vi "generate_DAC_voltages_V3_justMineZtrajectoryTest.vi"(7 "focus mode?":bool, 8 "derived values":T1, 9 "scan specification":T4={"x amplitude"=0, "x resolution (pixels)"=0, "x offset fly-forward (iterations)"=0, "x offset fly-back (iterations)"=0, "y resolution (nr. of lines)"=0, "y step size"=0, "iterations per pixel"=0, "number of frames"=0, "y offset (pixels)"=0, "number of y-brake lines  (before y-fly-back)"=0, "number y-brake lines (after y-fly-back)"=0, "number of y-fly-back steps"=8, "lines per z step"=0, "number of z/intensity tuples"=0, "number of repetitions (volumes or planes)"=0, "z step size derived"=0, "choose the beginning of z scan"=FALSE, "number of frames (settings)"=0, "FPGA trajectory?"=FALSE}, 10 "counter cluster in":T2, 11 "resonant trigger":bool) -> (0 "acquire?":bool, 1 "fly-back acquisition phase?":bool, 2 "counter cluster out":T2, 3 "DAC voltages":T3 {"ch6" max=4095 step=1; "ch5" max=4095 step=1; "ch4" max=4095 step=1; "ch3" max=4095 step=1; "ch2" max=4095 step=1; "ch1" max=4095 step=1; "ch0" max=4095 step=1})   [LabVIEW 2010]
uses:
  scan_specification_cluster.ctl
  common_typedefs/DAC_voltage_cluster.ctl
  counter_cluster.ctl
  derived_values_cluster.ctl
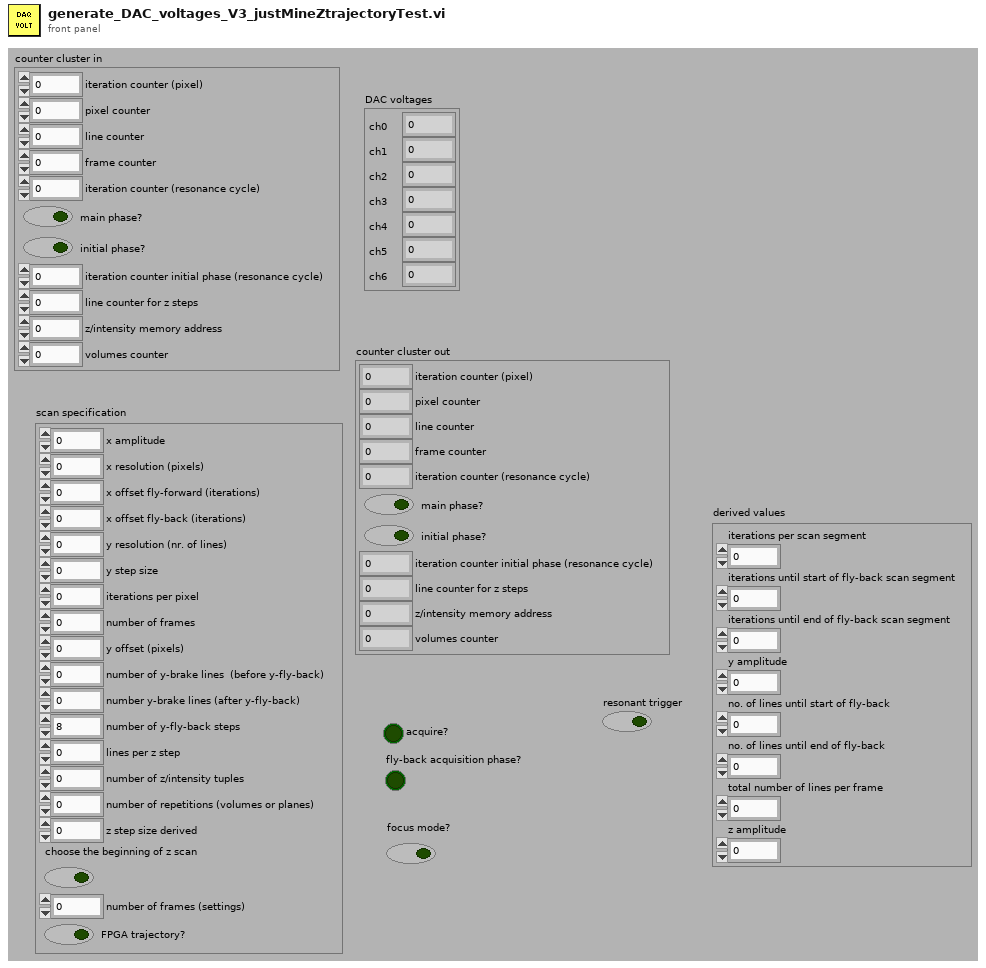
[diagram p1: front panel]
types:
  T1 = typedef "derived_values_cluster.ctl" = cluster{"iterations per scan segment":u16, "iterations until start of fly-back scan segment":u16, "iterations until end of fly-back scan segment":u16, "y amplitude":u16, "no. of lines until start of fly-back":u16, "no. of lines until end of fly-back":u16, "total number of lines per frame ":u16, "z amplitude":u16}
  T2 = typedef "counter_cluster.ctl" = cluster{"iteration counter (pixel)":u16, "pixel counter":u16, "line counter":u16, "frame counter":u16, "iteration counter (resonance cycle)":u16, "main phase?":bool, "initial phase?":bool, "iteration counter initial phase (resonance cycle)":u16, "line counter for z steps":u16, "z/intensity memory address":u32, "volumes counter":u16}
  T3 = typedef "DAC_voltage_cluster.ctl" = cluster{"ch0":u16, "ch1":i16, "ch2":i16, "ch3":u16, "ch4":u16, "ch5":u16, "ch6":u16}
  T4 = typedef "scan_specification_cluster.ctl" = cluster{"x amplitude":u16, "x resolution (pixels)":u16, "x offset fly-forward (iterations)":u16, "x offset fly-back (iterations)":u16, "y resolution (nr. of lines)":u16, "y step size":u16, "iterations per pixel":u16, "number of frames":i32, "y offset (pixels)":u16, "number of y-brake lines  (before y-fly-back)":u16, "number y-brake lines (after y-fly-back)":u16, "number of y-fly-back steps":u16, "lines per z step":u16, "number of z/intensity tuples":u16, "number of repetitions (volumes or planes)":i32, "z step size derived":u16, "choose the beginning of z scan":bool, "number of frames (settings)":i32, "FPGA trajectory?":bool}
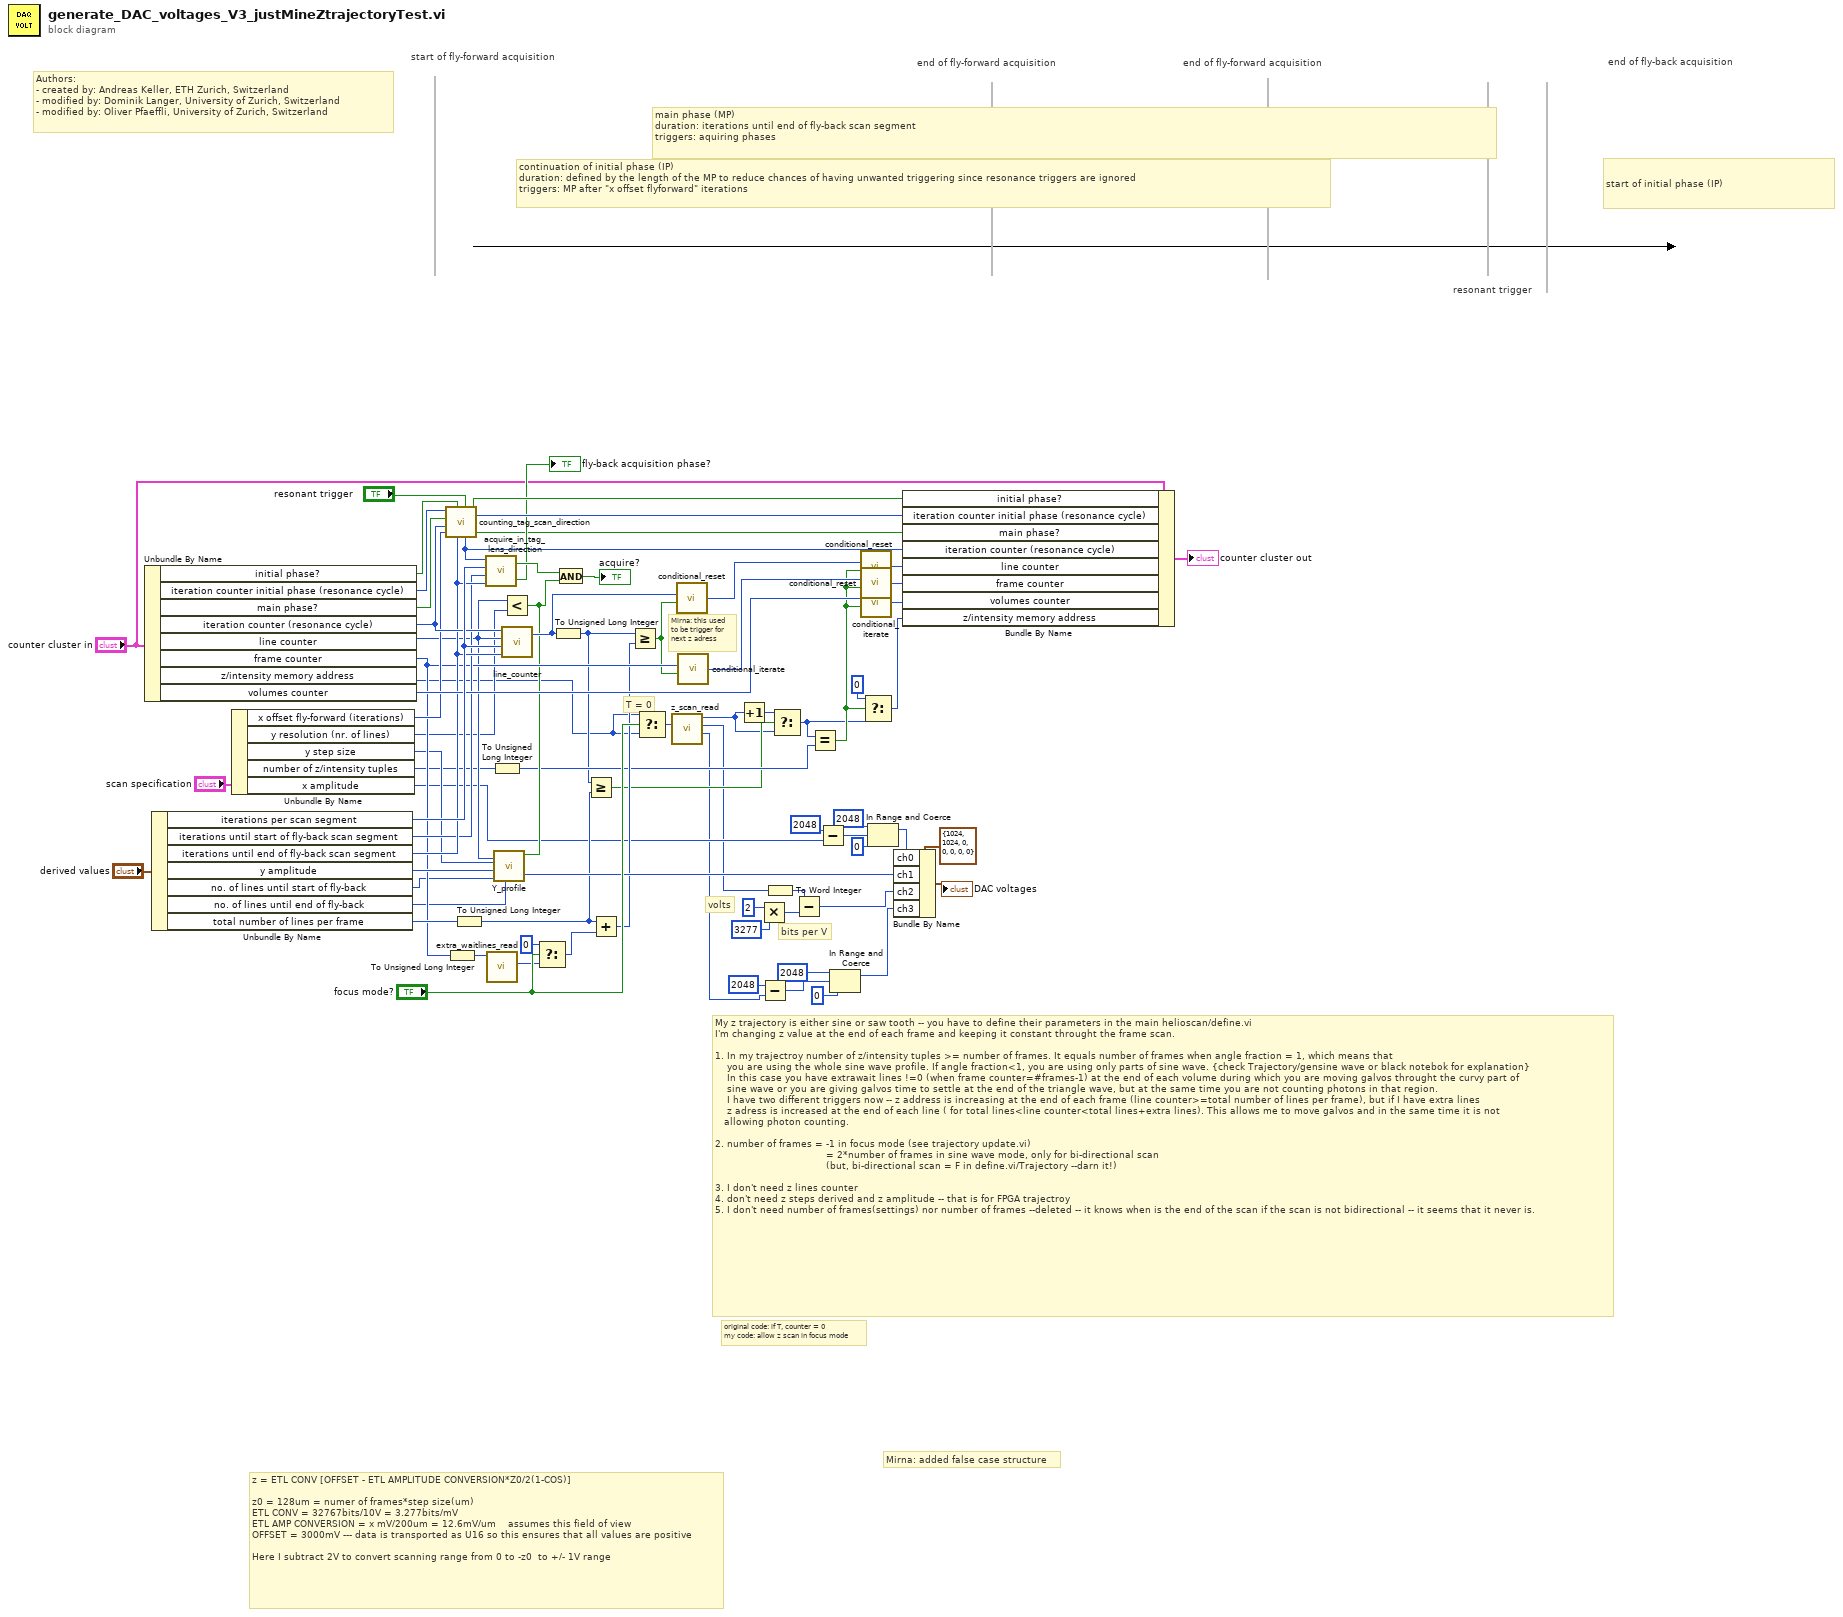
[diagram p0: block diagram]
diagram:
  # "bits per V"
  # "volts"
  # "Mirna: this used \nto be trigger for \nnext z adress"
  # "T = 0"
  # "My z trajectory is either sine or saw tooth -- you have to define their parameters in the main helioscan/define.vi\nI'm changing z value at the end of each frame and keeping it constant throught the frame scan.\n\n1. In my trajectroy number of z/intensity tuples >= number of frames. It equals number of frames when angle fraction = 1, which means that \n    you are using the whole sine wave profile. If angle fraction<1, you are using only parts of sine wave. {check Trajectory/gensine wave or black notebok for explanation}\n    In this case you have extrawait lines !=0 (when frame counter=#frames-1) at the end of each volume during which you are moving galvos throught the curvy part of\n    sine wave or you are giving galvos time to settle at the end of the triangle wave, but at the same time you are not counting photons in that region.\n    I have two different triggers now -- z address is increasing at the end of each frame (line counter>=total number of lines per frame), but if I have extra lines \n    z adress is increased at the end of each line ( for total lines<line counter<total lines+extra lines). This allows me to move galvos and in the same time it is not \n   allowing photon counting.\n   \n2. number of frames = -1 in focus mode (see trajectory update.vi)\n                                     = 2*number of frames in sine wave mode, only for bi-directional scan \n                                     (but, bi-directional scan = F in define.vi/Trajectory --darn it!)\n             \n3. I don't need z lines counter\n4. don't need z steps derived and z amplitude -- that is for FPGA trajectroy\n5. I don't need number of frames(settings) nor number of frames --deleted -- it knows when is the end of the scan if the scan is not bidirectional -- it seems that it never is."
  # "z = ETL CONV [OFFSET - ETL AMPLITUDE CONVERSION*Z0/2(1-COS)]\n\nz0 = 128um = numer of frames*step size(um)\nETL CONV = 32767bits/10V = 3.277bits/mV\nETL AMP CONVERSION = x mV/200um = 12.6mV/um    assumes this field of view\nOFFSET = 3000mV --- data is transported as U16 so this ensures that all values are positive\n\nHere I subtract 2V to convert scanning range from 0 to -z0  to +/- 1V range"
  # "original code: if T, counter = 0\nmy code: allow z scan in focus mode"
  # "Mirna: added false case structure"
  # "start of initial phase (IP)"
  # "continuation of initial phase (IP)\nduration: defined by the length of the MP to reduce chances of having unwanted triggering since resonance triggers are ignored\ntriggers: MP after \"x offset flyforward\" iterations"
  # "end of fly-back acquisition"
  # "end of fly-forward acquisition"
  # "end of fly-forward acquisition"
  # "start of fly-forward acquisition"
  # "main phase (MP)\nduration: iterations until end of fly-back scan segment\ntriggers: aquiring phases"
  # "resonant trigger"
  # "Authors: \n- created by: Andreas Keller, ETH Zurich, Switzerland\n- modified by: Dominik Langer, University of Zurich, Switzerland\n- modified by: Oliver Pfaeffli, University of Zurich, Switzerland"
  n1 = Unbundle By Name("counter cluster in") -> ("initial phase?"=w66:bool, "iteration counter initial phase (resonance cycle)"=w47:u16, "main phase?"=w57:bool, "iteration counter (resonance cycle)"=w46:u16, "line counter"=w39:u16, "frame counter"=w40:u16, "z/intensity memory address"=w15:u32, "volumes counter"=w59:u16)
  n2 = Unbundle By Name("derived values") -> ("iterations per scan segment"=w65:u16, "iterations until start of fly-back scan segment"=w44:u16, "iterations until end of fly-back scan segment"=w45:u16, "y amplitude"=w51:u16, "no. of lines until start of fly-back"=w37:u16, "no. of lines until end of fly-back"=w36:u16, "total number of lines per frame"=w53:u16)
  n3 = Unbundle By Name("scan specification") -> ("x offset fly-forward (iterations)"=w42:u16, "y resolution (nr. of lines)"=w33:u16, "y step size"=w38:u16, "number of z/intensity tuples"=w22:u16, "x amplitude"=w21:u16)
  n4 = call "counting_tag_scan_direction.vi"("resonant trigger"="resonant trigger", "initial phase?"=w66, "iteration counter initial phase (resonance cycle)"=w47, "main phase?"=w57, "iterations until end of fly-back scan segment"=w45, "iteration counter (resonance cycle)"=w46, "x offset fly-forward (iterations)"=w42) -> ("initial phase? OUT"=w49:bool, "iteration counter initial phase (resonance cycle) out"=w48:u16, "main phase? OUT"=w41:bool, "iteration counter (resonance cycle) out"=w28:u16)
  n5 = To Unsigned Long Integer(number=w40) -> (unsigned 32bit integer=w34:u32)
  n6 = To Unsigned Long Integer(number=w53) -> (unsigned 32bit integer=w24:u32)
  n7 = call "acquire_in_tag_lens_direction.vi"("iterations until end of fly-back scan segment"=w45, "iterations until start of fly-back scan segment"=w44, "iterations per scan segment"=w65, "iteration counter (resonance cycle) out"=w28) -> ("flyback phase?"=→"fly-back acquisition phase?":bool, "acquire during flyforward or flyback phase?"=w68:bool)
  n8 = call "extra_waitlines_read.vi"("address extra waitlines IN"=w34) -> ("extra waitline data"=w52:u32)  [unwired: 9 in, 1 out]
  n9 = To Unsigned Long Integer(number=w22) -> (unsigned 32bit integer=w19:u32)
  n10 = Less?(x=w39, y=w33) -> (x < y?=w26:bool)
  n11 = call "Y_profile.vi"("no. of lines until end of fly-back"=w36, "line counter"=w39, "no. of lines until start of fly-back"=w37, "y amplitude"=w51, "y step size"=w38, "y acquire? (line counter<number of lines)"=w26) -> ("y signal"=w56:i16)  [unwired: 1 in]
  n12 = call "line_counter.vi"("iterations until end of fly-back scan segment"=w45, "iterations per scan segment"=w65, "line counter in"=w39, "iteration counter (resonance cycle)"=w46) -> ("line counter out"=w29:u16)  [unwired: 1 out]
  n13 = Select(t=u32 0, s="focus mode?", f=w52) -> (s? t:f=w20:u32)
  n14 = To Unsigned Long Integer(number=w29) -> (unsigned 32bit integer=w18:u32)
  n15 = And(x=w68, y=w26) -> (x .and. y?=→"acquire?":bool)
  n16 = Greater Or Equal?(x=w18, y=w24) -> (x >= y?=w17:bool)
  n17 = Add(x=w24, y=w20) -> (x+y=w23:u32)
  n18 = Greater Or Equal?(x=w18, y=w23) -> (x >= y?=w25:bool)
  n19 = Select(t=w15, s="focus mode?", f=w15) -> (s? t:f=w6:u32)
  n20 = call "z_scan_read.vi"("address in"=w6) -> ("intensity"=w3:u16, "z-value"=w1:i16, "address out"=w5:u32)  [unwired: 8 in]
  n21 = call "conditional_reset.vi"("reset?"=w25, "number in"=w29) -> ("number out"=w62:u16)  [unwired: 4 in]
  n22 = call "conditional_iterate.vi"("iterate?"=w25, "number in"=w40) -> ("number out"=w54:u16)  [unwired: 4 in]
  n23 = Increment(x=w5) -> (x+1=w64:u32)
  n24 = Multiply(x=i16 2 ("y"), y=i16 3277) -> (x*y=w9:i16)
  n25 = Subtract(x=i16 2048, y=w3) -> (x-y=w14:u16)
  n26 = To Word Integer(number=w1) -> (16bit integer=w7:i16)
  n27 = Select(t=w64, s=w17, f=w5) -> (s? t:f=w16:u32)
  n28 = Subtract(x=w7, y=w9) -> (x-y=w2:i16)
  n29 = Equal?(x=w16, y=w19) -> (x = y?=w30:bool)
  n30 = Subtract(x=u16 2048, y=w21) -> (x-y=w72:u16)
  n31 = In Range and Coerce(upper limit=u16 2048, x=w14, lower limit=u16 0) -> (coerced(x)=w4:u16)  [unwired: 1 out]
  n32 = call "conditional_reset.vi"("reset?"=w30, "number in"=w62) -> ("number out"=w61:u16)  [unwired: 4 in]
  n33 = call "conditional_reset.vi"("reset?"=w30, "number in"=w54) -> ("number out"=w55:u16)  [unwired: 4 in]
  n34 = call "conditional_iterate.vi"("iterate?"=w30, "number in"=w59) -> ("number out"=w63:u16)  [unwired: 4 in]
  n35 = Select(t=u32 0, s=w30, f=w16) -> (s? t:f=w31:u32)
  n36 = In Range and Coerce(upper limit=u16 2048, x=w72, lower limit=u16 0) -> (coerced(x)=w71:u16)  [unwired: 1 out]
  n37 = Bundle By Name(cluster=T3 {"ch0"=1024, "ch1"=1024, "ch2"=0, "ch3"=0, "ch4"=0, "ch5"=0, "ch6"=0} ("DAC voltage"), "ch0"=w71, "ch1"=w56, "ch2"=w2, "ch3"=w4) -> (→"DAC voltages":T3)
  n38 = Bundle By Name(cluster="counter cluster in", "initial phase?"=w49, "iteration counter initial phase (resonance cycle)"=w48, "main phase?"=w41, "iteration counter (resonance cycle)"=w28, "line counter"=w61, "frame counter"=w55, "volumes counter"=w63, "z/intensity memory address"=w31) -> (→"counter cluster out":T2)
